vi "Start RFSG.vi"(0 "Path in":refnum<class "Scalar Path.lvclass">, 11 "error in (no error)":errorcluster) -> (4 "Path out":refnum<class "Scalar Path.lvclass">, 15 "error out":errorcluster)   [LabVIEW 2023, in "RFFixtureCharact.Public.lvlib" / "Scalar Path.lvclass"]
uses:
  Scalar Path.lvclass
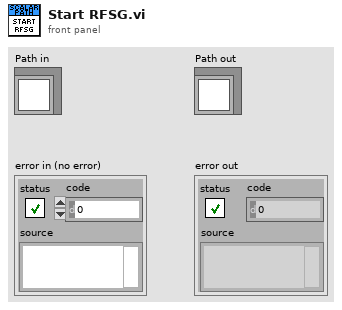
[diagram p1: front panel]
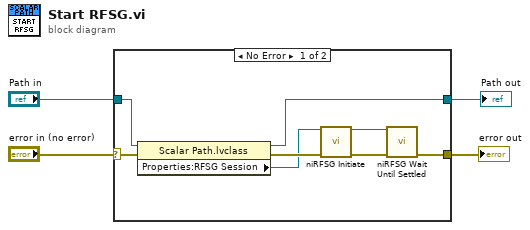
[diagram p0: block diagram]
diagram:
  n1 = case shown="No Error" "error in (no error)" {
    selector: "error in (no error)" -> [w11 w14]
    tunnel: [w6 w14] -> w3
    tunnel: [w10 w13] -> w1
    tunnel: "Path in" -> [w12 w13]
    frame No Error {
      n2 = property class="Scalar Path.lvclass"(reference=w12, error in=w11) -> (reference out=w10:refnum<class "Scalar Path.lvclass">, error out=w9:errorcluster, "Properties:RFSG Session"=w5:refnum<k15>)
      n3 = call <instrlib>:"niRFSG Initiate.vi"("instrument handle"=w5, "error in"=w9) -> ("instrument handle out"=w7:refnum<k15>, "error out"=w8:errorcluster)  [unwired: 12 in]
      n4 = call <instrlib>:"niRFSG Wait Until Settled.vi"("instrument handle"=w7, "error in"=w8) -> ("error out"=w6:errorcluster)  [unwired: 12 in, 1 out]
    }
    frame Error {
    }
  }
  "error out" <- w3
  "Path out" <- w1
